vi "Build Assert VI.vi"(8 "error in (no error)":errorcluster, 10 "Type":T4=enum."Double Float", 11 "VI Refnum":refnum<vi>) -> (0 "error out":errorcluster, 2 "Add Object":bool, 3 "appended path":path)   [LabVIEW 2016]
doc: "Dialog box which shows up and dynamically reconfigures during the process of creating a new assert"
uses:
  Numeric Operations.ctl
  <vilib>/Utility/Data Type/Type Definitions/Data Type.ctl
  String Operations.ctl
  FP UI References.ctl
  Assert Scripting Configuration.ctl
  <vilib>/Utility/Data Type/NI_Data Type.lvlib
panel:
  in  "I64 Comparison Value 2":i64 caption="Comparison Value"
  in  "I16 Comparison Value 2":i16 caption="Comparison Value"
  in  "I8 Comparison Value 2":i8 caption="Comparison Value"
  in  "U64 Comparison Value 2":u64 caption="Comparison Value"
  in  "U32 Comparison Value 2":u32 caption="Comparison Value"
  in  "U16 Comparison Value 2":u16 caption="Comparison Value"
  in  "U8 Comparison Value 2":u8 caption="Comparison Value"
  in  "U64 Comparison Value 1":u64 caption="Comparison Value"
  in  "U32 Comparison Value 1":u32 caption="Comparison Value"
  in  "U16 Comparison Value 1":u16 caption="Comparison Value"
  in  "U8 Comparison Value 1":u8 caption="Comparison Value"
  in  "I64 Comparison Value 1":i64 caption="Comparison Value"
  in  "I16 Comparison Value 1":i16 caption="Comparison Value"
  in  "I8 Comparison Value 1":i8 caption="Comparison Value"
  in  "EXT Comparison Value 2":ext caption="Comparison Value"
  in  "EXT Comparison Value 1":ext caption="Comparison Value"
  in  "SGL Comparison Value 2":sgl caption="Comparison Value"
  in  "SGL Comparison Value 1":sgl caption="Comparison Value"
  in  "Boolean Comparison Value":bool caption="Comparison Value"
  in  "String Operations":T1 caption="Operation"
  in  "Numeric Operation":T2="EQ" caption="Operation"
  in  "Default Failure Action":T3(ring)
  in  "Description":string
  in  "String Comparison Value":string caption="Comparison Value"
  in  "I32 Comparison Value 1":i32 caption="Comparison Value"
  in  "DBL Comparison Value 1":dbl caption="Comparison Value"
  in  "I32 Comparison Value 2":i32 caption="Comparison Value"
  in  "DBL Comparison Value 2":dbl caption="Comparison Value"
  in  "Comment":string
  in  "Assert Name":string
  in  "Create":bool
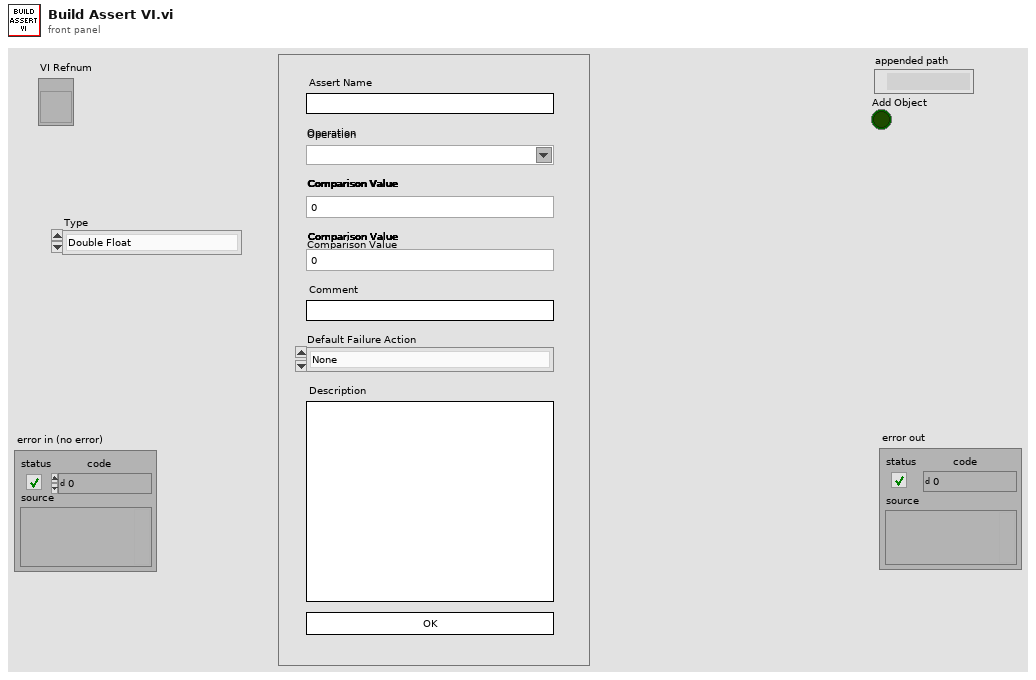
[diagram p1: front panel]
types:
  T1 = typedef "String Operations.ctl" = string
  T2 = typedef "Numeric Operations.ctl" = string
  T3 = enum16{"None", "Log To File", "Pause Execution", "Abort Execution"}
  T4 = typedef "NI_Data Type.lvlib/Data Type.ctl" = enum8{"Invalid Type", "Void", "I8", "I16", "I32", "I64", "U8", "U16", "U32", "U64", "Single Float", "Double Float", "Extended Float", "Single Complex", "Double Complex", "Extended Complex", "Enum U8", "Enum U16", "Enum U32", "Enum U64", "Single Float With Unit", "Double Float With Unit", "Extended Float With Unit", "Single Complex with Unit", "Double Complex with Unit", "Extended Complex with Unit", "Boolean", "String", "Path", "Picture", "Tag", "Array", "Cluster", "Variant", "LV Variant", "Waveform", "Timestamp", "Digital Waveform", "Digital Data", "ExpressData", "Refnum", "External Data", "VI", "Poly VI", "LabVIEW Class Instance", "Fixed Point"}
  T5 = typedef "FP UI References.ctl" = cluster{"String Comparison Value":refnum<vi>, "DBL Comparison Value 1":refnum<vi>, "DBL Comparison Value 2":refnum<vi>, "I32 Comparison Value 1":refnum<vi>, "I32 Comparison Value 2":refnum<vi>, "String Operation":refnum<vi>, "Numeric Operation":refnum<vi>, "Boolean Comparison Value":refnum<vi>, "I8 Comparison Value 1":refnum<vi>, "I8 Comparison Value 2":refnum<vi>, "I16 Comparison Value 1":refnum<vi>, "I16 Comparison Value 2":refnum<vi>, "I64 Comparison Value 1":refnum<vi>, "I64 Comparison Value 2":refnum<vi>, "U16 Comparison Value 1":refnum<vi>, "U8 Comparison Value 1":refnum<vi>, "U8 Comparison Value 2":refnum<vi>, "U16 Comparison Value 2":refnum<vi>, "U32 Comparison Value 1":refnum<vi>, "U32 Comparison Value 2":refnum<vi>, "U64 Comparison Value 1":refnum<vi>, "U64 Comparison Value 2":refnum<vi>, "SGL Comparison Value 1":refnum<vi>, "SGL Comparison Value 2":refnum<vi>, "EXT Comparison Value 1":refnum<vi>, "EXT Comparison Value 2":refnum<vi>}
  T6 = typedef "Assert Scripting Configuration.ctl" = cluster{"Assert Name":string, "Comment":string, "Numeric Operation":string, "Type":T4, "String Operation":string, "DBL Comparison Value 1":dbl, "DBL Comparison Value 2":dbl, "I32 Comparison Value 1":i32, "I32 Comparison Value 2":i32, "Creator":string, "Creation Timestamp":timestamp, "String Comparison Value":string, "Description":string, "Default Failure Action":enum16{"None", "Log To File", "Pause Execution", "Abort Execution"}, "Boolean Comparison Value":bool, "I8 Comparison Value 1":i8, "I8 Comparison Value 2":i8, "I16 Comparison Value 1":i16, "I16 Comparison Value 2":i16, "I64 Comparison Value 1":i64, "I64 Comparison Value 2":i64, "U8 Comparison Value 1":u8, "U8 Comparison Value 2":u8, "U16 Comparison Value 1":u16, "U16 Comparison Value 2":u16, "U32 Comparison Value 1":u32, "U32 Comparison Value 2":u32, "U64 Comparison Value 1":u64, "U64 Comparison Value 2":u64, "EXT Comparison Value 1":ext, "EXT Comparison Value 2":ext, "SGL Comparison Value 1":sgl, "SGL Comparison Value 2":sgl}
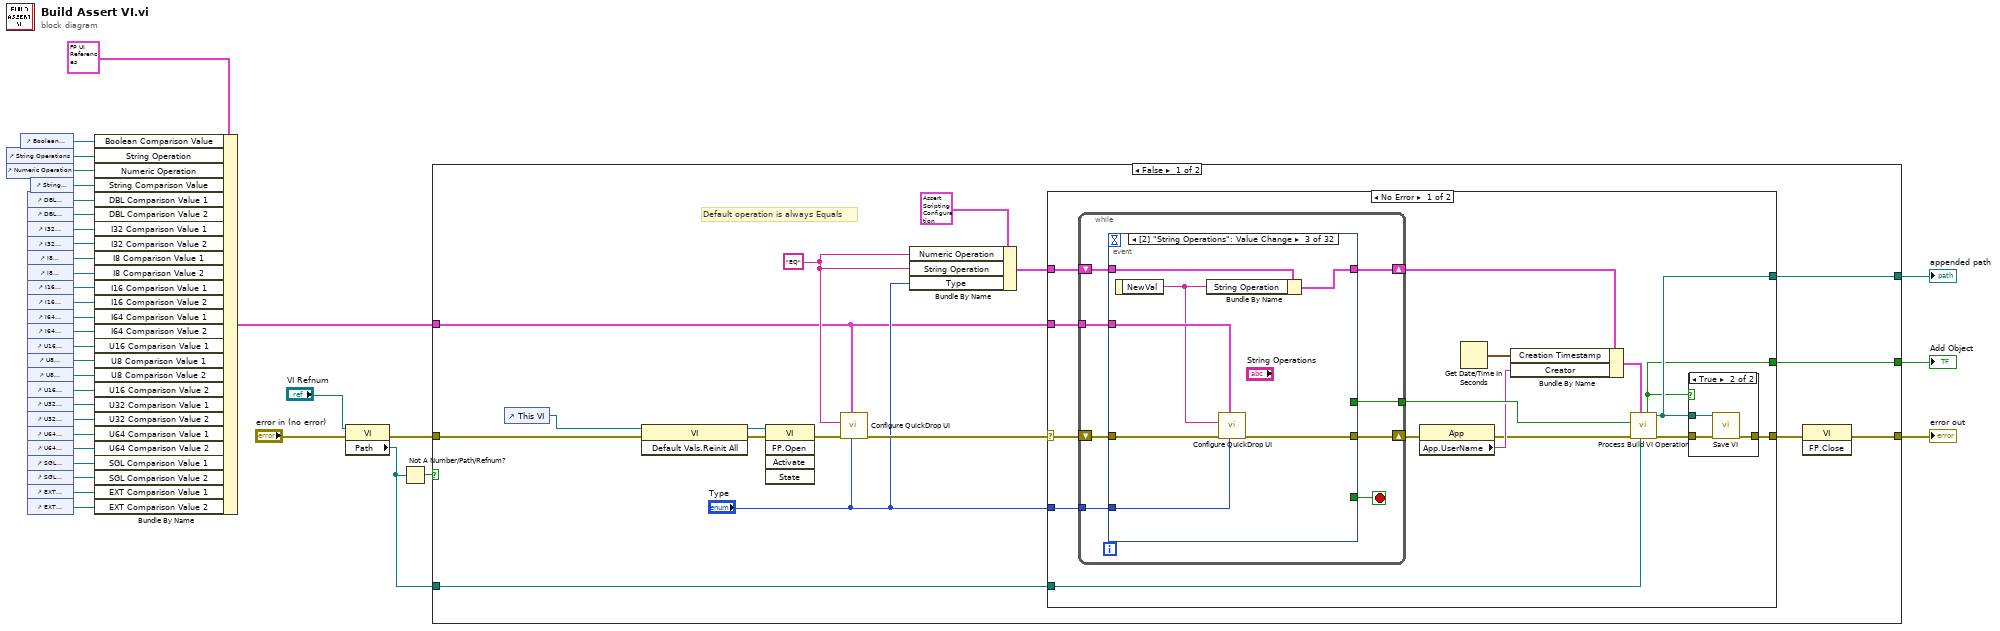
[diagram p0: block diagram]
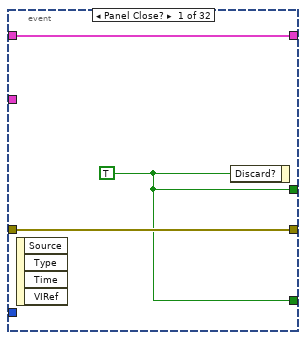
[diagram p3: hidden frame]
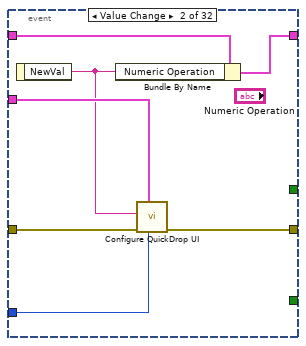
[diagram p4: hidden frame]
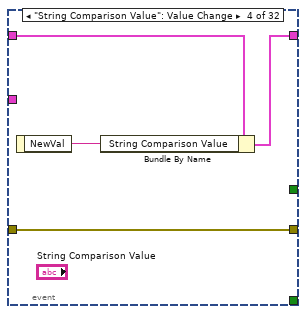
[diagram p5: hidden frame]
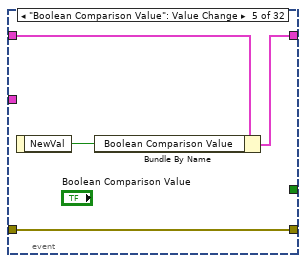
[diagram p6: hidden frame]
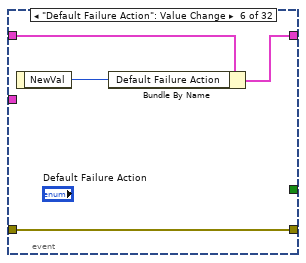
[diagram p7: hidden frame]
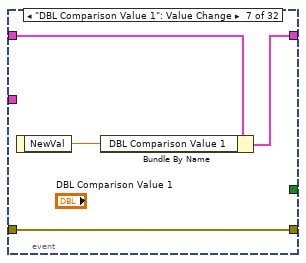
[diagram p8: hidden frame]
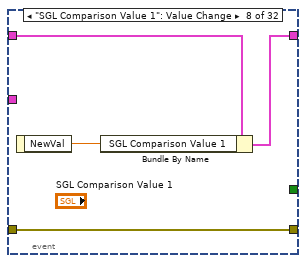
[diagram p9: hidden frame]
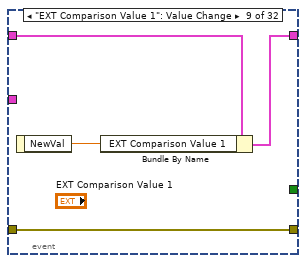
[diagram p10: hidden frame]
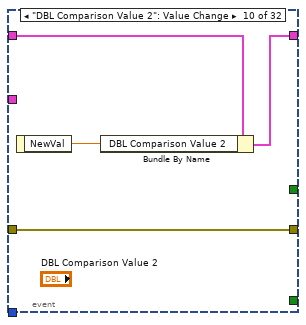
[diagram p11: hidden frame]
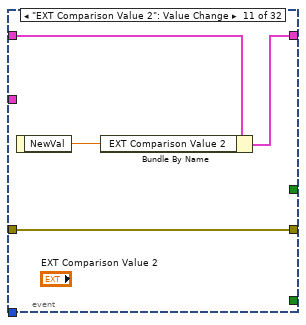
[diagram p12: hidden frame]
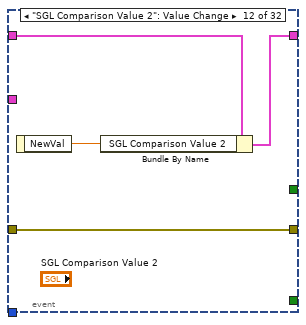
[diagram p13: hidden frame]
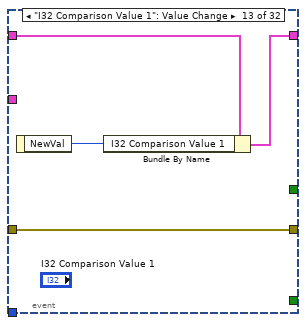
[diagram p14: hidden frame]
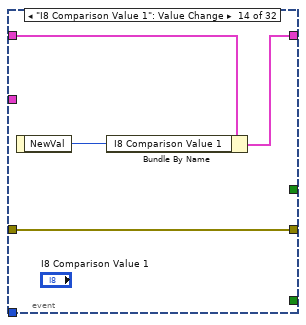
[diagram p15: hidden frame]
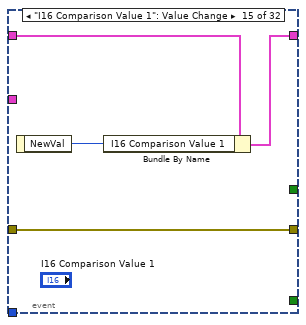
[diagram p16: hidden frame]
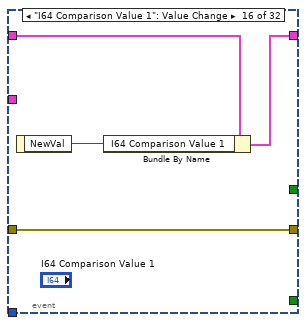
[diagram p17: hidden frame]
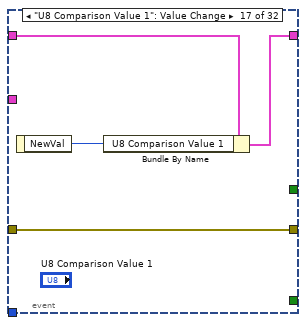
[diagram p18: hidden frame]
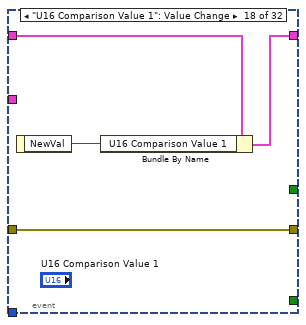
[diagram p19: hidden frame]
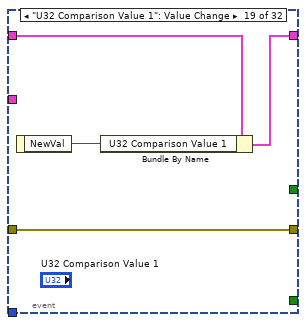
[diagram p20: hidden frame]
diagram:
  n1 = control-ref of="String Operations"() -> (w27:refnum<vi>)
  n2 = control-ref of="Numeric Operation"() -> (w26:refnum<vi>)
  n3 = control-ref of="Boolean Comparison Value"() -> (w28:refnum<vi>)
  n4 = control-ref of="DBL Comparison Value 1"() -> (w23:refnum<vi>)
  n5 = control-ref of="DBL Comparison Value 2"() -> (w22:refnum<vi>)
  n6 = control-ref of="I32 Comparison Value 1"() -> (w21:refnum<vi>)
  n7 = control-ref of="I32 Comparison Value 2"() -> (w20:refnum<vi>)
  n8 = control-ref of="I8 Comparison Value 1"() -> (w17:refnum<vi>)
  n9 = control-ref of="I8 Comparison Value 2"() -> (w6:refnum<vi>)
  n10 = control-ref of="I16 Comparison Value 1"() -> (w16:refnum<vi>)
  n11 = control-ref of="I16 Comparison Value 2"() -> (w5:refnum<vi>)
  n12 = control-ref of="I64 Comparison Value 1"() -> (w15:refnum<vi>)
  n13 = control-ref of="I64 Comparison Value 2"() -> (w4:refnum<vi>)
  n14 = control-ref of="U16 Comparison Value 1"() -> (w13:refnum<vi>)
  n15 = control-ref of="U8 Comparison Value 1"() -> (w14:refnum<vi>)
  n16 = control-ref of="U8 Comparison Value 2"() -> (w10:refnum<vi>)
  n17 = control-ref of="U16 Comparison Value 2"() -> (w9:refnum<vi>)
  n18 = control-ref of="U32 Comparison Value 1"() -> (w12:refnum<vi>)
  n19 = control-ref of="U32 Comparison Value 2"() -> (w8:refnum<vi>)
  n20 = control-ref of="U64 Comparison Value 1"() -> (w11:refnum<vi>)
  n21 = control-ref of="U64 Comparison Value 2"() -> (w7:refnum<vi>)
  n22 = control-ref of="SGL Comparison Value 1"() -> (w3:refnum<vi>)
  n23 = control-ref of="SGL Comparison Value 2"() -> (w18:refnum<vi>)
  n24 = control-ref of="EXT Comparison Value 1"() -> (w2:refnum<vi>)
  n25 = control-ref of="EXT Comparison Value 2"() -> (w1:refnum<vi>)
  n26 = control-ref of="String Comparison Value"() -> (w24:refnum<vi>)
  n27 = Bundle By Name(cluster=T5 {"String Comparison Value"=refnum, "DBL Comparison Value 1"=refnum, "DBL Comparison Value 2"=refnum, "I32 Comparison Value 1"=refnum, "I32 Comparison Value 2"=refnum, "String Operation"=refnum, "Numeric Operation"=refnum, "Boolean Comparison Value"=refnum, "I8 Comparison Value 1"=refnum, "I8 Comparison Value 2"=refnum, "I16 Comparison Value 1"=refnum, "I16 Comparison Value 2"=refnum, "I64 Comparison Value 1"=refnum, "I64 Comparison Value 2"=refnum, "U16 Comparison Value 1"=refnum, "U8 Comparison Value 1"=refnum, "U8 Comparison Value 2"=refnum, "U16 Comparison Value 2"=refnum, "U32 Comparison Value 1"=refnum, "U32 Comparison Value 2"=refnum, "U64 Comparison Value 1"=refnum, "U64 Comparison Value 2"=refnum, "SGL Comparison Value 1"=refnum, "SGL Comparison Value 2"=refnum, "EXT Comparison Value 1"=refnum, "EXT Comparison Value 2"=refnum}, "Boolean Comparison Value"=w28, "String Operation"=w27, "Numeric Operation"=w26, "String Comparison Value"=w24, "DBL Comparison Value 1"=w23, "DBL Comparison Value 2"=w22, "I32 Comparison Value 1"=w21, "I32 Comparison Value 2"=w20, "I8 Comparison Value 1"=w17, "I8 Comparison Value 2"=w6, "I16 Comparison Value 1"=w16, "I16 Comparison Value 2"=w5, "I64 Comparison Value 1"=w15, "I64 Comparison Value 2"=w4, "U16 Comparison Value 1"=w13, "U8 Comparison Value 1"=w14, "U8 Comparison Value 2"=w10, "U16 Comparison Value 2"=w9, "U32 Comparison Value 1"=w12, "U32 Comparison Value 2"=w8, "U64 Comparison Value 1"=w11, "U64 Comparison Value 2"=w7, "SGL Comparison Value 1"=w3, "SGL Comparison Value 2"=w18, "EXT Comparison Value 1"=w2, "EXT Comparison Value 2"=w1) -> (w19:T5)
  n28 = property class="VI"(reference="VI Refnum", error in="error in (no error)") -> (error out=w32:errorcluster, "Path"=w35:path)  [unwired: 1 out]
  n29 = Not A Number/Path/Refnum?(number/path/refnum=w35) -> (NaN/Path/Refnum?=w34:bool)
  n30 = case shown="False" w34 {
    tunnel: w35 -> [w52 _]
    tunnel: w32 -> [w51 w215]
    tunnel: [w49 w215] -> w31
    tunnel: [w45 _] -> w30
    tunnel: [w44 _] -> w29
    tunnel: w19 -> [w37 _]
    frame False {
      w39 = "EQ" ("Numeric Operation")
      # "Default operation is always Equals"
      n31 = control-ref of="This VI"() -> (w46:refnum<vi>)
      n32 = invoke class="VI" method="Default Vals.Reinit All"(reference=w46, error in=w51) -> (reference out=w47:refnum<vi>, error out=w48:errorcluster)  [unwired: 1 in, 1 out]
      n33 = invoke class="VI" method="FP.Open"(reference=w47, error in=w48) -> (error out=w50:errorcluster)  [unwired: 3 in, 4 out]
      n34 = call "Configure QuickDrop UI.vi"("Type"="Type", "FP UI References"=w37, "error in (no error)"=w50, "Operation"=w39) -> ("error out"=w43:errorcluster)  [unwired: 7 in]
      n35 = Bundle By Name(cluster=T6 {"Assert Name"="", "Comment"="", "Numeric Operation"="", "Type"=enum."Double Float", "String Operation"="", "DBL Comparison Value 1"=0.0, "DBL Comparison Value 2"=0.0, "I32 Comparison Value 1"=0, "I32 Comparison Value 2"=0, "Creator"="", "Creation Timestamp"=timestamp(0 s since 1904-01-01), "String Comparison Value"="", "Description"="", "Default Failure Action"=enum."None", "Boolean Comparison Value"=FALSE, "I8 Comparison Value 1"=0, "I8 Comparison Value 2"=0, "I16 Comparison Value 1"=0, "I16 Comparison Value 2"=0, "I64 Comparison Value 1"=0, "I64 Comparison Value 2"=0, "U8 Comparison Value 1"=0, "U8 Comparison Value 2"=0, "U16 Comparison Value 1"=0, "U16 Comparison Value 2"=0, "U32 Comparison Value 1"=0, "U32 Comparison Value 2"=0, "U64 Comparison Value 1"=0, "U64 Comparison Value 2"=0, "EXT Comparison Value 1"=0.0, "EXT Comparison Value 2"=0.0, "SGL Comparison Value 1"=0.0, "SGL Comparison Value 2"=0.0}, "Numeric Operation"=w39, "String Operation"=w39, "Type"="Type") -> (w41:T6)
      n36 = case shown="No Error" w43 {
        selector: w43 -> [w67 w213]
        tunnel: w52 -> [w63 _]
        tunnel: [w55 _] -> w40
        tunnel: [w54 _] -> w45
        tunnel: [w53 _] -> w44
        tunnel: w41 -> [w66 _]
        tunnel: w37 -> [w62 _]
        tunnel: "Type" -> [w61 _]
        frame No Error {
          n37 = while {
            tunnel: [w80] -> w64
            shift-right: [w79] -> w57
            shift-left: w67 -> [w78]
            shift-right: [w75] -> w65
            shift-left: w66 -> [w76]
            tunnel: w62 -> [w74]
            tunnel: w61 -> [w73]
            stop <- w77 stop-if-true
            n38 = event shown="[2] \"String Operations\": Value Change" {
              selector: _ -> [_ _ _ _ _ _ _ _ _ _ _ _ _ _ _ _ _ _ _ _ _ _ _ _ _ _ _ _ _ _ _ _]
              dyn-events: _ -> [_ _ _ _ _ _ _ _ _ _ _ _ _ _ _ _ _ _ _ _ _ _ _ _ _ _ _ _ _ _ _ _]
              timeout: _ -> [_ _ _ _ _ _ _ _ _ _ _ _ _ _ _ _ _ _ _ _ _ _ _ _ _ _ _ _ _ _ _ _]
              tunnel: [w82 _ _ _ _ _ _ _ _ _ _ _ _ _ _ _ _ _ _ _ _ _ _ _ _ _ _ _ _ _ _ _] -> w80
              tunnel: w78 -> [w83 w89 w96 w100 w104 w108 w112 w116 w120 w124 w128 w132 w136 w140 w144 w148 w152 w156 w160 w164 w168 w172 w176 w180 w184 w188 w192 w196 w198 w202 w206 w212]
              tunnel: [w83 w87 w94 w100 w104 w108 w112 w116 w120 w124 w128 w132 w136 w140 w144 w148 w152 w156 w160 w164 w168 w172 w176 w180 w184 w188 w192 w196 w198 w202 w206 w212] -> w79
              tunnel: [w82 _ _ _ _ _ _ _ _ _ _ _ _ _ _ _ _ _ _ _ _ _ _ _ _ _ _ _ _ _ _ TRUE] -> w77
              tunnel: w76 -> [w81 w90 w97 w101 w105 w109 w113 w117 w121 w125 w129 w133 w137 w141 w145 w149 w153 w157 w161 w165 w169 w173 w177 w181 w185 w189 w193 w197 w201 w205 w209 w210]
              tunnel: [w81 w88 w95 w99 w103 w107 w111 w115 w119 w123 w127 w131 w135 w139 w143 w147 w151 w155 w159 w163 w167 w171 w175 w179 w183 w187 w191 w195 w200 w204 w208 w210] -> w75
              tunnel: w74 -> [_ w86 w93 _ _ _ _ _ _ _ _ _ _ _ _ _ _ _ _ _ _ _ _ _ _ _ _ _ _ _ _ _]
              tunnel: w73 -> [_ w84 w91 _ _ _ _ _ _ _ _ _ _ _ _ _ _ _ _ _ _ _ _ _ _ _ _ _ _ _ _ _]
              event Panel Close? {
                w82 = TRUE ("Discard?")
                n39 = event-data() -> ()  [unwired: 1 in, 4 out]
                n40 = event-data("Discard?"=w82) -> ()  [unwired: 1 in, 1 out]
              }
              event Value Change {
                n41 = event-data() -> ("NewVal"=w85:T2)  [unwired: 1 in]
                n42 = Bundle By Name(cluster=w90, "Numeric Operation"=w85) -> (w88:T6)
                n43 = call "Configure QuickDrop UI.vi"("Type"=w84, "FP UI References"=w86, "error in (no error)"=w89, "Operation"=w85) -> ("error out"=w87:errorcluster)  [unwired: 7 in]
              }
              event Value Change {
                n44 = event-data() -> ("NewVal"=w92:T1)  [unwired: 1 in]
                n45 = Bundle By Name(cluster=w97, "String Operation"=w92) -> (w95:T6)
                n46 = call "Configure QuickDrop UI.vi"("Type"=w91, "FP UI References"=w93, "error in (no error)"=w96, "Operation"=w92) -> ("error out"=w94:errorcluster)  [unwired: 7 in]
              }
              event "String Comparison Value": Value Change {
                n47 = event-data() -> ("NewVal"=w98:string)  [unwired: 1 in]
                n48 = Bundle By Name(cluster=w101, "String Comparison Value"=w98) -> (w99:T6)
              }
              event "Boolean Comparison Value": Value Change {
                n49 = event-data() -> ("NewVal"=w102:bool)  [unwired: 1 in]
                n50 = Bundle By Name(cluster=w105, "Boolean Comparison Value"=w102) -> (w103:T6)
              }
              event "Default Failure Action": Value Change {
                n51 = event-data() -> ("NewVal"=w106:T3)  [unwired: 1 in]
                n52 = Bundle By Name(cluster=w109, "Default Failure Action"=w106) -> (w107:T6)
              }
              event "DBL Comparison Value 1": Value Change {
                n53 = event-data() -> ("NewVal"=w110:dbl)  [unwired: 1 in]
                n54 = Bundle By Name(cluster=w113, "DBL Comparison Value 1"=w110) -> (w111:T6)
              }
              event "SGL Comparison Value 1": Value Change {
                n55 = event-data() -> ("NewVal"=w114:sgl)  [unwired: 1 in]
                n56 = Bundle By Name(cluster=w117, "SGL Comparison Value 1"=w114) -> (w115:T6)
              }
              event "EXT Comparison Value 1": Value Change {
                n57 = event-data() -> ("NewVal"=w118:ext)  [unwired: 1 in]
                n58 = Bundle By Name(cluster=w121, "EXT Comparison Value 1"=w118) -> (w119:T6)
              }
              event "DBL Comparison Value 2": Value Change {
                n59 = event-data() -> ("NewVal"=w122:dbl)  [unwired: 1 in]
                n60 = Bundle By Name(cluster=w125, "DBL Comparison Value 2"=w122) -> (w123:T6)
              }
              event "EXT Comparison Value 2": Value Change {
                n61 = event-data() -> ("NewVal"=w126:ext)  [unwired: 1 in]
                n62 = Bundle By Name(cluster=w129, "EXT Comparison Value 2"=w126) -> (w127:T6)
              }
              event "SGL Comparison Value 2": Value Change {
                n63 = event-data() -> ("NewVal"=w130:sgl)  [unwired: 1 in]
                n64 = Bundle By Name(cluster=w133, "SGL Comparison Value 2"=w130) -> (w131:T6)
              }
              event "I32 Comparison Value 1": Value Change {
                n65 = event-data() -> ("NewVal"=w134:i32)  [unwired: 1 in]
                n66 = Bundle By Name(cluster=w137, "I32 Comparison Value 1"=w134) -> (w135:T6)
              }
              event "I8 Comparison Value 1": Value Change {
                n67 = event-data() -> ("NewVal"=w138:i8)  [unwired: 1 in]
                n68 = Bundle By Name(cluster=w141, "I8 Comparison Value 1"=w138) -> (w139:T6)
              }
              event "I16 Comparison Value 1": Value Change {
                n69 = event-data() -> ("NewVal"=w142:i16)  [unwired: 1 in]
                n70 = Bundle By Name(cluster=w145, "I16 Comparison Value 1"=w142) -> (w143:T6)
              }
              event "I64 Comparison Value 1": Value Change {
                n71 = event-data() -> ("NewVal"=w146:i64)  [unwired: 1 in]
                n72 = Bundle By Name(cluster=w149, "I64 Comparison Value 1"=w146) -> (w147:T6)
              }
              event "U8 Comparison Value 1": Value Change {
                n73 = event-data() -> ("NewVal"=w150:u8)  [unwired: 1 in]
                n74 = Bundle By Name(cluster=w153, "U8 Comparison Value 1"=w150) -> (w151:T6)
              }
              event "U16 Comparison Value 1": Value Change {
                n75 = event-data() -> ("NewVal"=w154:u16)  [unwired: 1 in]
                n76 = Bundle By Name(cluster=w157, "U16 Comparison Value 1"=w154) -> (w155:T6)
              }
              event "U32 Comparison Value 1": Value Change {
                n77 = event-data() -> ("NewVal"=w158:u32)  [unwired: 1 in]
                n78 = Bundle By Name(cluster=w161, "U32 Comparison Value 1"=w158) -> (w159:T6)
              }
              event "U64 Comparison Value 1": Value Change {
                n79 = event-data() -> ("NewVal"=w162:u64)  [unwired: 1 in]
                n80 = Bundle By Name(cluster=w165, "U64 Comparison Value 1"=w162) -> (w163:T6)
              }
              event "I32 Comparison Value 2": Value Change {
                n81 = event-data() -> ("NewVal"=w166:i32)  [unwired: 1 in]
                n82 = Bundle By Name(cluster=w169, "I32 Comparison Value 2"=w166) -> (w167:T6)
              }
              event "U8 Comparison Value 2": Value Change {
                n83 = event-data() -> ("NewVal"=w170:u8)  [unwired: 1 in]
                n84 = Bundle By Name(cluster=w173, "U8 Comparison Value 2"=w170) -> (w171:T6)
              }
              event "U16 Comparison Value 2": Value Change {
                n85 = event-data() -> ("NewVal"=w174:u16)  [unwired: 1 in]
                n86 = Bundle By Name(cluster=w177, "U16 Comparison Value 2"=w174) -> (w175:T6)
              }
              event "U32 Comparison Value 2": Value Change {
                n87 = event-data() -> ("NewVal"=w178:u32)  [unwired: 1 in]
                n88 = Bundle By Name(cluster=w181, "U32 Comparison Value 2"=w178) -> (w179:T6)
              }
              event "U64 Comparison Value 2": Value Change {
                n89 = event-data() -> ("NewVal"=w182:u64)  [unwired: 1 in]
                n90 = Bundle By Name(cluster=w185, "U64 Comparison Value 2"=w182) -> (w183:T6)
              }
              event "I8 Comparison Value 2": Value Change {
                n91 = event-data() -> ("NewVal"=w186:i8)  [unwired: 1 in]
                n92 = Bundle By Name(cluster=w189, "I8 Comparison Value 2"=w186) -> (w187:T6)
              }
              event "I16 Comparison Value 2": Value Change {
                n93 = event-data() -> ("NewVal"=w190:i16)  [unwired: 1 in]
                n94 = Bundle By Name(cluster=w193, "I16 Comparison Value 2"=w190) -> (w191:T6)
              }
              event "I64 Comparison Value 2": Value Change {
                n95 = event-data() -> ("NewVal"=w194:i64)  [unwired: 1 in]
                n96 = Bundle By Name(cluster=w197, "I16 Comparison Value 2"=w194) -> (w195:T6)
              }
              event "Assert Name": Value Change {
                n97 = event-data() -> ("NewVal"=w199:string)  [unwired: 1 in]
                n98 = Bundle By Name(cluster=w201, "Assert Name"=w199) -> (w200:T6)
              }
              event "Comment": Value Change {
                n99 = event-data() -> ("NewVal"=w203:string)  [unwired: 1 in]
                n100 = Bundle By Name(cluster=w205, "Comment"=w203) -> (w204:T6)
              }
              event "Description": Value Change {
                n101 = event-data() -> ("NewVal"=w207:string)  [unwired: 1 in]
                n102 = Bundle By Name(cluster=w209, "Description"=w207) -> (w208:T6)
              }
              event "Create": Value Change {
                n103 = event-data() -> ()  [unwired: 1 in, 1 out]
              }
            }
          }
          n104 = property class="App"(error in=w57) -> (error out=w56:errorcluster, "App.UserName"=w58:string)  [unwired: 1 in, 1 out]
          n105 = Get Date/Time In Seconds() -> (seconds since 1Jan1904=w59:timestamp)
          n106 = Bundle By Name(cluster=w65, "Creation Timestamp"=w59, "Creator"=w58) -> (w60:T6)
          n107 = call "Process Build VI Operation.vi"("Caller VI Path"=w63, "Assert Scripting Configuration"=w60, "error in (no error)"=w56, "Discard?"=w64) -> ("error out"=w68:errorcluster, "Assert VI Path"=w54:path, "Valid Configuration"=w53:bool)  [unwired: 5 in]
          n108 = case shown="True" w53 {
            tunnel: w68 -> [w69 w72]
            tunnel: [w69 w71] -> w55
            tunnel: w54 -> [_ w70]
            frame False {
            }
            frame True {
              n109 = call "Save VI.vi"("error in (no error)"=w72, "Assert VI Path"=w70) -> ("error out"=w71:errorcluster)  [unwired: 9 in]
            }
          }
        }
        frame Error {
          n110 = call <vilib>:"Simple Error Handler.vi"("error in (no error)"=w213) -> ()  [unwired: 4 in, 5 out]
        }
      }
      n111 = invoke class="VI" method="FP.Close"(error in=w40) -> (error out=w49:errorcluster)  [unwired: 2 in, 2 out]
    }
    frame True {
      n112 = One Button Dialog(message="Invalid VI Path - No Assert statements can be created\nSave VI") -> ()  [unwired: 1 in, 1 out]
    }
  }
  "error out" <- w31
  "appended path" <- w30
  "Add Object" <- w29
